vi "7_MultiplicationTable.vi"() -> ()   [LabVIEW 2015]
panel:
  out "multiplication table":i32[][](array[numeric])
  # "1"
  # "2"
  # "3"
  # "4"
  # "5"
  # "6"
  # "7"
  # "8"
  # "9"
  # "10"
  # "11"
  # "12"
  # "1"
  # "2"
  # "3"
  # "4"
  # "5"
  # "6"
  # "7"
  # "8"
  # "9"
  # "10"
  # "11"
  # "12"
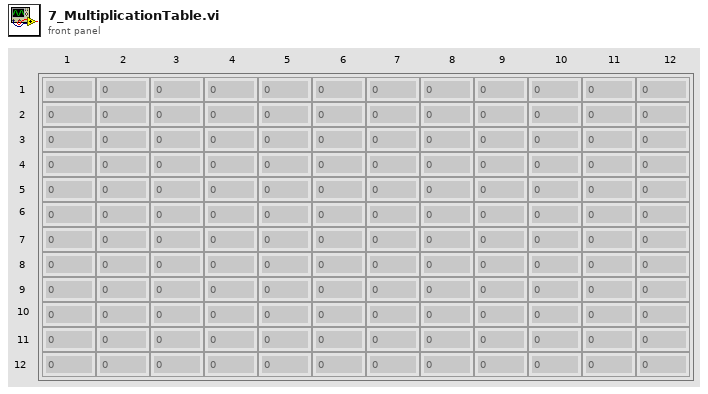
[diagram p1: front panel]
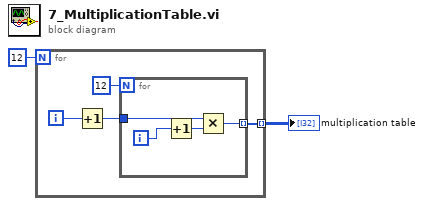
[diagram p0: block diagram]
diagram:
  n1 = for {
    N: 12 -> [_]
    tunnel: [w3] -> w1 mode=indexing
    i -> [w6]
    n2 = Increment(x=w6) -> (x+1=w5:i32)
    n3 = for {
      N: 12 -> [_]
      tunnel: w5 -> [w10]
      tunnel: [w8] -> w3 mode=indexing
      i -> [w9]
      n4 = Increment(x=w9) -> (x+1=w7:i32)
      n5 = Multiply(x=w10, y=w7) -> (x*y=w8:i32)
    }
  }
  "multiplication table" <- w1
